vi "Periodic Tasks.vi"(8 "error in (no error)":errorcluster) -> ()   [LabVIEW 2018]
doc: "This VI runs in parallel to other tasks. It can contain as many user-defined periodic loops as you need. These can carry out PID or other sorts of timed response."
uses:
  TrapezoidalMotionProfile/Constraints.ctl
  <vilib>/Rock Robotics/WPI/ThirdParty/Phoenix-LabVIEW/Motor Controller/Controls/CTRE_Phoenix_MotorControl_ControlMode.ctl
  Support Code/Wrist Angle.vi
  <vilib>/Rock Robotics/Network Tables/NT Read String.vi
  <vilib>/Rock Robotics/Network Tables/NT Write String.vi
  <vilib>/Rock Robotics/WPI/ThirdParty/Phoenix-LabVIEW/Motor Controller/Get/CTRE_Phoenix_MotorController_GetSelectedSensorData.vi
  TrapezoidalMotionProfile/TrapezoidalProfile.lvclass
  <vilib>/Rock Robotics/WPI/ThirdParty/REV Robotics/SPARK MAX/Typedef/Spark MAX Control Type.ctl
  <extravilib>/ChannelInstances/Tag-class'TrapezoidalProfile'.lvlib
  TrapezoidalMotionProfile/State.ctl
  <vilib>/Rock Robotics/WPI/ThirdParty/Phoenix-LabVIEW/Motor Controller/Get/CTRE_Phoenix_MotorController_GetVoltage.vi
  Robot Global Data.vi
panel:
  in  "Elevator Constraints":T1
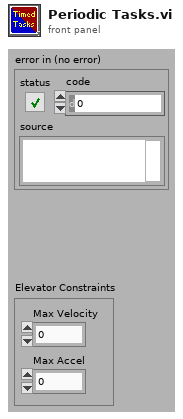
[diagram p1: front panel]
types:
  T1 = typedef "TrapezoidalProfile.lvclass/Constraints.ctl" = cluster{"Max Velocity":dbl, "Max Accel":dbl}
  T2 = typedef "WPI_MotorControlDeviceRef.ctl" = cluster{"DeviceStatus":errorcluster, "Type":T3, "PWM":cluster{"PWM Channel":T4, "DeadBand":T5}, "CAN":cluster{"Device Number":u8, "SetOutput VI Ref":variant, "GetOutput VI Ref":variant, "Enable VI Ref":variant, "Disable VI Ref":variant, "Data":variant}, "Invert":bool, "DIO PWM":cluster{"PWM \"Enable\" Channel":T4, "DIOChannel":T6, "PWM Rate":dbl}}
  T3 = typedef "WPI_MotorControlType.ctl" = enum16{"PWM", "CAN", "DIO PWM"}
  T4 = typedef "FPGA_DIOPWMChannel.ctl" = enum8{"PWM 0", "PWM 1", "PWM 2", "PWM 3", "PWM 4", "PWM 5", "PWM 6", "PWM 7", "PWM 8", "PWM 9", "PWM MXP 0", "PWM MXP 1", "PWM MXP 2", "PWM MXP 3", "PWM MXP 4", "PWM MXP 5", "PWM MXP 6", "PWM MXP 7", "PWM MXP 8", "PWM MXP 9", "Invalid"}
  T5 = typedef "WPI_PWMDeadband.ctl" = cluster{"Name":string, "maxPositivePwm":i32, "minPositivePwm":i32, "centerPwm":i32, "maxNegativePwm":i32, "minNegativePwm":i32, "angularRange":u16}
  T6 = typedef "FPGA_DIOChannel.ctl" = enum8{"DIO 0", "DIO 1", "DIO 2", "DIO 3", "DIO 4", "DIO 5", "DIO 6", "DIO 7", "DIO 8", "DIO 9", "DIO MXP 0", "DIO MXP 1", "DIO MXP 2", "DIO MXP 3", "DIO MXP 4", "DIO MXP 5", "DIO MXP 6", "DIO MXP 7", "DIO MXP 8", "DIO MXP 9", "DIO MXP 10", "DIO MXP 11", "DIO MXP 12", "DIO MXP 13", "DIO MXP 14", "DIO MXP 15", "SPI Port CS1", "SPI Port CS2", "SPI Port CS3", "SPI Port MISO", "SPI Port MOSI", "Invalid"}
  T7 = typedef "CTRE_Phoenix_MotorControl_ControlMode.ctl" = u16
  T8 = typedef "Spark MAX Control Type.ctl" = enum16{"Percent VBus", "Voltage", "Velocity", "Position", "Smart Motion", "Current", "Smart Velocity"}
  T9 = typedef "TrapezoidalProfile.lvclass/State.ctl" = cluster{"Position (u)":dbl, "Velocity (u/s)":dbl}
  T10 = typedef "Tag-class'TrapezoidalProfile'.lvlib/))Channel.ctl" = refnum<queue>
  T11 = enum16{"DemandType_Neutral", "DemandType_AuxPID", "DemandType_ArbitraryFeedForward"}
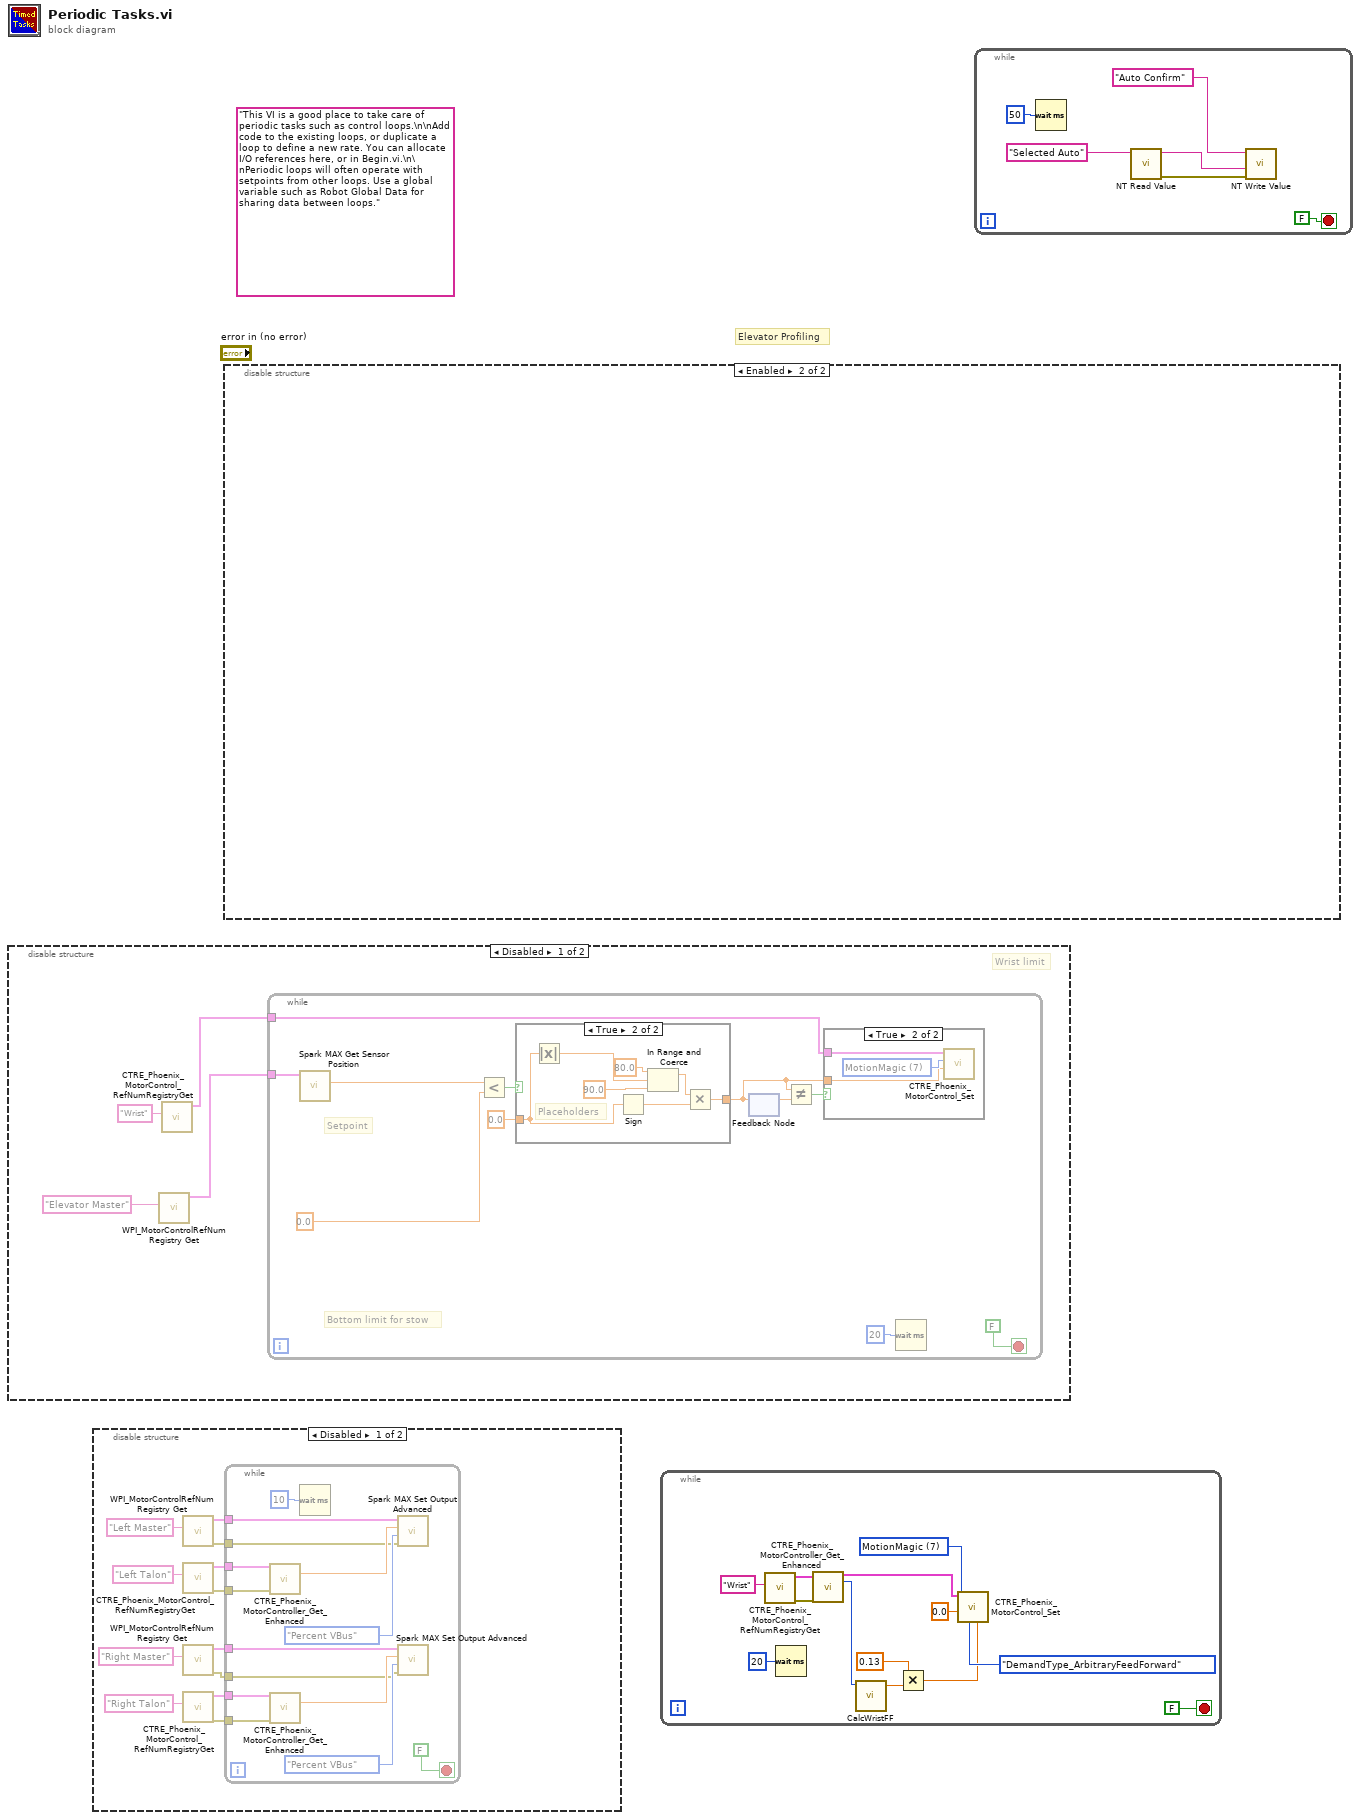
[diagram p0: block diagram]
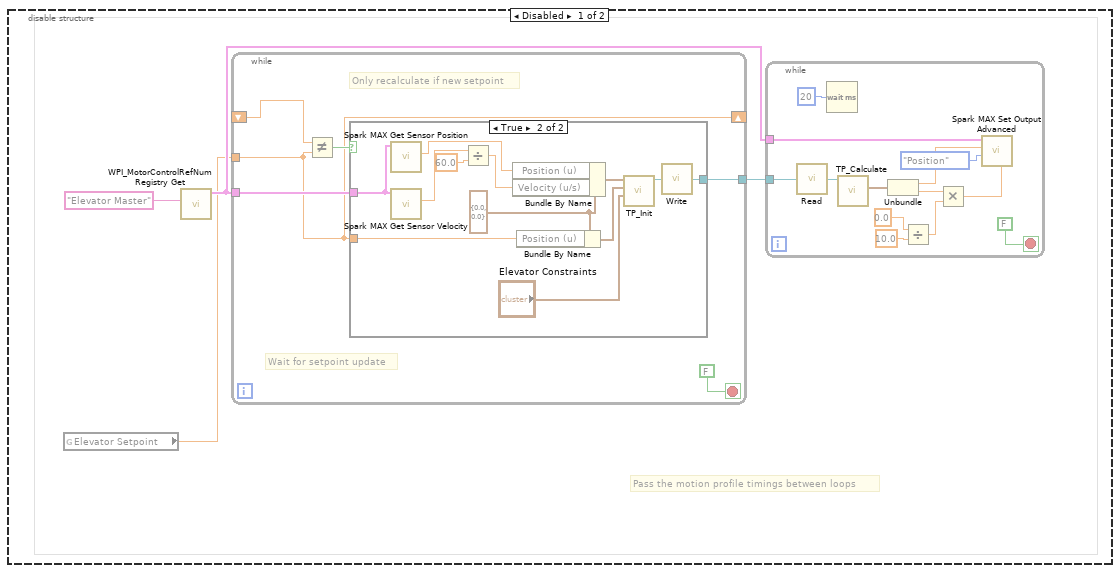
[diagram p3: hidden frame]
diagram:
  (unwired) "This VI is a good place to take care of periodic tasks such as control loops.\n\nAdd code to the existing loops, or duplicate a loop to define a new rate. You can allocate I/O references here, or in Begin.vi.\n\nPeriodic loops will often operate with setpoints from other loops. Use a global variable such as Robot Global Data for sharing data between loops."
  # "Elevator Profiling"
  n1 = disable-structure shown="Disabled" {
    frame Disabled {
      # "Wrist limit"
      n2 = call <vilib>:"WPI_MotorControlRefNum Registry Get.vi"("refnum name"="Elevator Master") -> ("MotorControlDevRef"=w2:T2)  [unwired: 9 in, 1 out]
      n3 = call <vilib>:"CTRE_Phoenix_MotorControl_RefNumRegistryGet.vi"("refnum name"="Wrist") -> ("PhoenixMotorControlDevRef"=w1:T2)  [unwired: 9 in, 1 out]
      n4 = while {
        tunnel: w2 -> [w14]
        tunnel: w1 -> [w9]
        stop <- FALSE stop-if-true
        # "Setpoint"
        # "Bottom limit for stow"
        n5 = call <vilib>:"Spark MAX Get Sensor Position.vi"("MotorControlDevRef in"=w14) -> ("Sensor Position"=w13:dbl)  [unwired: 7 in, 3 out]
        n6 = Less?(x=w13, y=0.0) -> (x < y?=w11:bool)
        n7 = case shown="True" w11 {
          tunnel: 0.0 -> [w19 w24]
          tunnel: [w19 w21] -> w5
          frame False {
          }
          frame True {
            # "Placeholders"
            n8 = Absolute Value(x=w24) -> (abs(x)=w23:dbl)
            n9 = Sign(1:w24) -> (0:w20:dbl)
            n10 = In Range and Coerce(upper limit=80.0, x=w23, lower limit=90.0) -> (coerced(x)=w22:dbl)  [unwired: 1 out]
            n11 = Multiply(x=w22, y=w20) -> (x*y=w21:dbl)
          }
        }
        n12 = feedback-in #1(w5) -> ()
        n13 = feedback #1() -> (w6:dbl)  [unwired: 1 in]
        n14 = Not Equal?(x=w5, y=w6) -> (x != y?=w7:bool)
        n15 = case shown="True" w7 {
          tunnel: w9 -> [_ w18]
          tunnel: w5 -> [_ w16]
          frame False {
          }
          frame True {
            w17 = T7 7 items=["PercentOutput"=0, "Position"=1, "Velocity"=2, "Current"=3, "Follower"=5, "MotionProfile"=6, "MotionMagic"=7, "MotionProfileArc"=10, "Disabled"=15] ("Control Mode")
            n16 = call <vilib>:"CTRE_Phoenix_MotorControl_Set.vi"("Output"=w16, "Control Mode"=w17, "PhoenixMotorControlDevRef"=w18) -> ()  [unwired: 7 in, 2 out]
          }
        }
        n17 = Wait (ms)(milliseconds to wait=u32 20) -> ()  [unwired: 1 out]
      }
    }
    frame Enabled {
    }
  }
  n18 = disable-structure shown="Disabled" {
    frame Disabled {
      n19 = call <vilib>:"WPI_MotorControlRefNum Registry Get.vi"("refnum name"="Left Master") -> ("error out"=w34:errorcluster, "MotorControlDevRef"=w35:T2)  [unwired: 9 in]
      n20 = call <vilib>:"CTRE_Phoenix_MotorControl_RefNumRegistryGet.vi"("refnum name"="Left Talon") -> ("error out"=w33:errorcluster, "PhoenixMotorControlDevRef"=w38:T2)  [unwired: 9 in]
      n21 = call <vilib>:"WPI_MotorControlRefNum Registry Get.vi"("refnum name"="Right Master") -> ("error out"=w32:errorcluster, "MotorControlDevRef"=w36:T2)  [unwired: 9 in]
      n22 = call <vilib>:"CTRE_Phoenix_MotorControl_RefNumRegistryGet.vi"("refnum name"="Right Talon") -> ("error out"=w31:errorcluster, "PhoenixMotorControlDevRef"=w37:T2)  [unwired: 9 in]
      n23 = while {
        tunnel: w38 -> [w51]
        tunnel: w37 -> [w50]
        tunnel: w36 -> [w49]
        tunnel: w35 -> [w44]
        tunnel: w34 -> [w42]
        tunnel: w33 -> [w41]
        tunnel: w32 -> [w40]
        tunnel: w31 -> [w39]
        stop <- FALSE stop-if-true
        n24 = call-poly <vilib>:"CTRE_Phoenix_MotorController_Get_Enhanced.vi"("PhoenixMotorControlDevRef"=w51, "error in"=w41) -> ("Percent Output"=w46:dbl)  [unwired: 9 in, 4 out]
        n25 = call-poly <vilib>:"CTRE_Phoenix_MotorController_Get_Enhanced.vi"("PhoenixMotorControlDevRef"=w50, "error in"=w39) -> ("Percent Output"=w47:dbl)  [unwired: 9 in, 4 out]
        n26 = Wait (ms)(milliseconds to wait=u32 10) -> ()  [unwired: 1 out]
        n27 = call <vilib>:"Spark MAX Set Output Advanced.vi"("error in (no error)"=w42, "Control Mode"=Spark_MAX_Control_Type."Percent VBus", "Setpoint"=w46, "MotorControlDevRef"=w44) -> ()  [unwired: 6 in, 2 out]
        n28 = call <vilib>:"Spark MAX Set Output Advanced.vi"("error in (no error)"=w40, "Control Mode"=Spark_MAX_Control_Type."Percent VBus", "Setpoint"=w47, "MotorControlDevRef"=w49) -> ()  [unwired: 6 in, 2 out]
      }
    }
    frame Enabled {
    }
  }
  n29 = disable-structure shown="Enabled" {
    frame Disabled {
      # "Pass the motion profile timings between loops"
      n30 = global read "Robot Global Data.vi" "Elevator Setpoint"() -> (w53:dbl)
      n31 = call <vilib>:"WPI_MotorControlRefNum Registry Get.vi"("refnum name"="Elevator Master") -> ("MotorControlDevRef"=w55:T2)  [unwired: 9 in, 1 out]
      n32 = while {
        tunnel: [w61] -> w56
        shift-right: [w57] -> _
        shift-left: _ -> [w59]
        tunnel: w55 -> [w58]
        tunnel: w53 -> [w57]
        stop <- FALSE stop-if-true
        # "Only recalculate if new setpoint"
        # "Wait for setpoint update"
        n33 = Not Equal?(x=w59, y=w57) -> (x != y?=w62:bool)
        n34 = case shown="True" w62 {
          tunnel: [_ w73] -> w61
          tunnel: w57 -> [_ w72]
          tunnel: w58 -> [_ w69]
          frame False {
          }
          frame True {
            w63 = T9 {"Position (u)"=0.0, "Velocity (u/s)"=0.0} ("Unprofiled Goal")
            n35 = call <vilib>:"Spark MAX Get Sensor Position.vi"("MotorControlDevRef in"=w69) -> ("Sensor Position"=w68:dbl)  [unwired: 7 in, 3 out]
            n36 = call <vilib>:"Spark MAX Get Sensor Velocity.vi"("MotorControlDevRef in"=w69) -> ("Sensor Velocity"=w66:dbl)  [unwired: 7 in, 3 out]
            n37 = Divide(x=w66, y=60.0) -> (x/y=w65:dbl)
            n38 = Bundle By Name(cluster=w63, "Position (u)"=w68, "Velocity (u/s)"=w65) -> (w64:T9)
            n39 = Bundle By Name(cluster=w63, "Position (u)"=w72) -> (w71:T9)
            n40 = call "TP_Init.vi"("Constraints"="Elevator Constraints", "Unprofiled Goal"=w71, "Initial"=w64) -> ("TrapezoidalProfile out"=w74:refnum<class "TrapezoidalProfile.lvclass">)  [unwired: 7 in, 1 out]
            n41 = call <extravilib>:"Write.vi"("element"=w74) -> ("channel"=w73:T10)  [unwired: 1 out]
          }
        }
      }
      n42 = while {
        tunnel: w55 -> [w75]
        tunnel: w56 -> [w77]
        stop <- FALSE stop-if-true
        n43 = call <extravilib>:"Read.vi"("channel"=w77) -> ("element"=w76:refnum<class "TrapezoidalProfile.lvclass">)  [unwired: 1 in, 1 out]
        n44 = Wait (ms)(milliseconds to wait=u32 20) -> ()  [unwired: 1 out]
        n45 = call "TP_Calculate.vi"("TrapezoidalProfile in"=w76) -> ("Output"=w85:T9)  [unwired: 8 in, 2 out]
        n46 = Unbundle(w85) -> ("Position (u)"=w84:dbl, "Velocity (u/s)"=w80:dbl)
        n47 = Divide(x=0.0, y=10.0) -> (x/y=w81:dbl)
        n48 = Multiply(x=w80, y=w81) -> (x*y=w79:dbl)
        n49 = call <vilib>:"Spark MAX Set Output Advanced.vi"("Arbitrary Feed Forward (0)"=w79, "Control Mode"=Spark_MAX_Control_Type."Position", "Setpoint"=w84, "MotorControlDevRef"=w75) -> ()  [unwired: 6 in, 2 out]
      }
    }
    frame Enabled {
    }
  }
  n50 = while {
    stop <- FALSE stop-if-true
    w100 = T7 7 items=["PercentOutput"=0, "Position"=1, "Velocity"=2, "Current"=3, "Follower"=5, "MotionProfile"=6, "MotionMagic"=7, "MotionProfileArc"=10, "Disabled"=15] ("Control Mode")
    n51 = call <vilib>:"CTRE_Phoenix_MotorControl_RefNumRegistryGet.vi"("refnum name"="Wrist") -> ("error out"=w95:errorcluster, "PhoenixMotorControlDevRef"=w96:T2)  [unwired: 9 in]
    n52 = Wait (ms)(milliseconds to wait=u32 20) -> ()  [unwired: 1 out]
    n53 = call-poly <vilib>:"CTRE_Phoenix_MotorController_Get_Enhanced.vi"("PhoenixMotorControlDevRef"=w96, "error in"=w95) -> ("PhoenixMotorControlDevRef"=w90:T2, "Position (Raw Sensor Units)"=w94:i32)  [unwired: 10 in, 2 out]
    n54 = call "CalcWristFF.vi"("Ticks (from vertical)"=w94) -> ("Vert Force Scalar"=w93:dbl)  [unwired: 10 in]
    n55 = Multiply(x=0.13, y=w93) -> (x*y=w91:dbl)
    n56 = call <vilib>:"CTRE_Phoenix_MotorControl_Set.vi"("Demand1"=w91, "DemandType"=T11."DemandType_ArbitraryFeedForward", "Output"=0.0, "Control Mode"=w100, "PhoenixMotorControlDevRef"=w90) -> ()  [unwired: 5 in, 2 out]
  }
  n57 = while {
    stop <- FALSE stop-if-true
    n58 = Wait (ms)(milliseconds to wait=u32 50) -> ()  [unwired: 1 out]
    n59 = call-poly <vilib>:"NT Read Value.vi"("Name"="Selected Auto") -> ("error out"=w101:errorcluster, "String"=w105:string)  [unwired: 9 in]
    n60 = call-poly <vilib>:"NT Write Value.vi"("error in"=w101, "String"=w105, "Name"="Auto Confirm") -> ()  [unwired: 8 in, 1 out]
  }
